vi "Configure Trigger Level.vi"(7 "Trigger Level (0.001 V)":dbl=0.001 format="%#_4g", 8 "error in (no error)":errorcluster, 9 "Trigger Slope (0:Positive)":i32(ring) items=["Positive", "Negative"], 10 "Channel (1:Channel 1)":i32(ring)=1 items=["Channel 1"=1, "Channel 2"=2], 11 "VISA resource name":refnum<visa-resource-name>) -> (0 "error out":errorcluster, 3 "VISA resource name out":refnum<visa-resource-name>)   [LabVIEW 2020, in "Template - Counter.lvlib"]
doc: "Configures the Trigger Level. If needed, this VI should be called after the <b>Configure Measurement</b> VI."
uses:
  <instrlib>/_Template - Counter/Template - Counter.lvlib
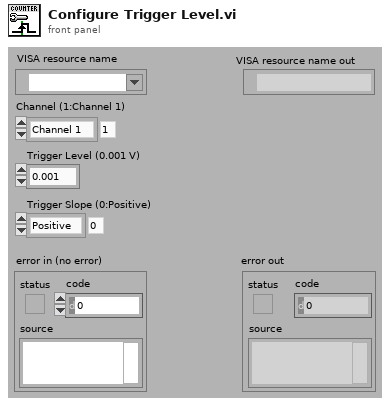
[diagram p1: front panel]
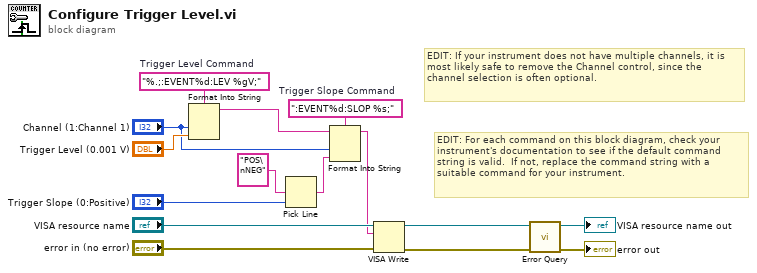
[diagram p0: block diagram]
diagram:
  w12 = ":EVENT%d:SLOP %s;"  # Trigger Slope Command
  w13 = "%.;:EVENT%d:LEV %gV;"  # Trigger Level Command
  # "EDIT: If your instrument does not have multiple channels, it is most likely safe to remove the Channel control, since the channel selection is often optional."
  # "EDIT: For each command on this block diagram, check your instrument's documentation to see if the default command string is valid.  If not, replace the command string with a suitable command for your instrument."
  n1 = Format Into String(format string=w13, "Channel (1:Channel 1)", "Trigger Level (0.001 V)") -> (resulting string=w2:string)  [unwired: 2 in, 1 out]
  n2 = Pick Line(multi-line string="POS\nNEG", line index="Trigger Slope (0:Positive)") -> (output string=w4:string)  [unwired: 1 in]
  n3 = Format Into String(format string=w12, initial string=w2, "Channel (1:Channel 1)", w4) -> (resulting string=w3:string)  [unwired: 1 in, 1 out]
  n4 = VISA Write(VISA resource name="VISA resource name", write buffer=w3, error in (no error)="error in (no error)") -> (VISA resource name out=w11:refnum<visa-resource-name>, error out=w9:errorcluster)  [unwired: 1 out]
  n5 = call <instrlib>:"Error Query.vi"("error in (no error)"=w9, "VISA resource name"=w11) -> ("error out"=→"error out":errorcluster, "VISA resource name out"=→"VISA resource name out":refnum<visa-resource-name>)  [unwired: 6 in, 2 out]
